vi "Receive Message.vi"(6 "priority":i32, 10 "Machine d'état in":refnum<class "Machine d'état.lvclass">, 11 "Message in":refnum<class "Message.lvclass">) -> (0 "error out":errorcluster, 2 "Actor out":refnum<class "Actor.lvclass">)   [LabVIEW 2020, in "Machine d'état.lvlib" / "Machine d'état.lvclass"]
doc: "This VI should be overriden ONLY if you are creating a proxy actor for remote transmission. If you are, override this VI to transmit the received message to a new destination, maintaining the given priority."
uses:
  <vilib>/ActorFramework/Message/Message.lvclass
  <vilib>/ActorFramework/Actor/Actor.lvclass
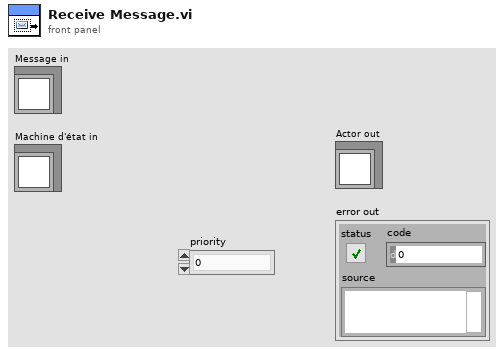
[diagram p1: front panel]
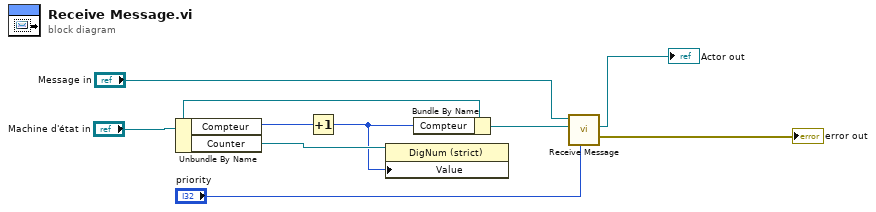
[diagram p0: block diagram]
diagram:
  n1 = Unbundle By Name("Machine d'état in") -> ("Compteur"=w5:u8, "Counter"=w4:refnum<vi>)
  n2 = Increment(x=w5) -> (x+1=w3:u8)
  n3 = property class="DigNum (strict)"(reference=w4, "Value"=w3) -> ()  [unwired: 1 in, 2 out]
  n4 = Bundle By Name(cluster="Machine d'état in", "Compteur"=w3) -> (w1:refnum<class "Machine d'état.lvclass">)
  n5 = call-parent "Receive Message.vi"("priority"="priority", "Actor in"=w1, "Message in"="Message in") -> ("error out"=→"error out":errorcluster, "Actor out"=→"Actor out":refnum<class "Actor.lvclass">)  [unwired: 7 in]
